vi "NF87XX.ProcPeriodic.vi"(0 "i ref in":refnum<vi>, 3 "ms timeout (100)":i32=100, 5 "error in (no error)":errorcluster) -> (14 "i ref out":refnum<vi>, 17 "timed out":bool, 19 "error out":errorcluster)   [LabVIEW 2014, in "NF87XX.lvlib"]
doc: "This method serves to periodically do things like reading values from the HW. Methods that should be executed periodically should be called from THIS methode. Add code here."
uses:
  NF87XX.lvlib
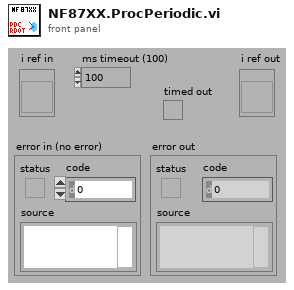
[diagram p1: front panel]
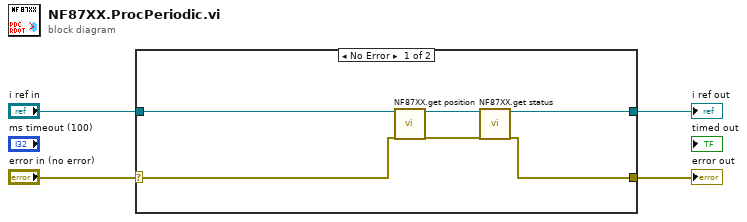
[diagram p0: block diagram]
diagram:
  n1 = case shown="No Error" "error in (no error)" {
    selector: "error in (no error)" -> [w9 w11]
    tunnel: "i ref in" -> [w10 w12]
    tunnel: [w5 w12] -> w3
    tunnel: [w7 w11] -> w2
    frame No Error {
      n2 = call "NF87XX.get position.vi"("i ref in"=w10, "error in (no error)"=w9) -> ("i ref out"=w6:refnum<vi>, "error out"=w8:errorcluster)  [unwired: 15 in, 1 out]
      n3 = call "NF87XX.get status.vi"("i ref in"=w6, "error in (no error)"=w8) -> ("i ref out"=w5:refnum<vi>, "error out"=w7:errorcluster)  [unwired: 15 in, 1 out]
    }
    frame Error {
    }
  }
  "error out" <- w2
  "i ref out" <- w3
